vi "Prepare Log.vi"(8 "error in (no error)":errorcluster, 10 "Log":string, 11 "Log Manager Module in":refnum<class "Log Manager Module.lvclass">) -> (0 "error out":errorcluster, 3 "Log Manager Module out":refnum<class "Log Manager Module.lvclass">)   [LabVIEW 2020, in "VolatusData.lvlib" / "Log Manager Module.lvclass"]
uses:
  Log Manager Module.lvclass
  C:/dev/lv20CE/relink/lv-volatus/Volatus/Module/Module.lvclass
  Prep State.ctl
  Log Manager Module.lvclass/Log Manager Module.ctl
  <vilib>/Utility/miscctls.llb/LVMapReplaceAction.ctl
  Prep Info.ctl
  Log Preparer Module/Log Preparer Module.lvclass
  VolatusData.lvlib
  C:/dev/lv20CE/relink/lv-volatus/VolatusData/Log Manager Module/Log Manager Module.lvclass
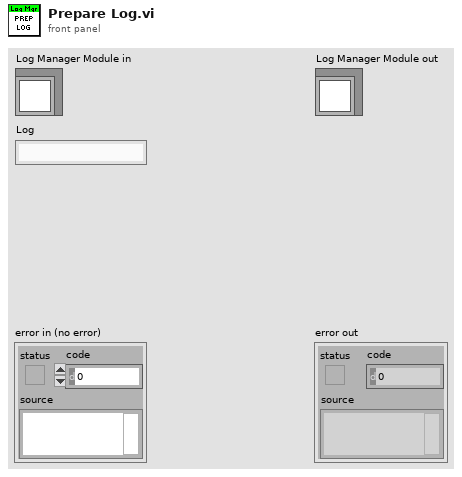
[diagram p1: front panel]
types:
  T1 = typedef "VolatusData.lvlib/Prep State.ctl" = enum16{"Unknown", "In Progress", "Success", "Failed"}
  T2 = typedef "VolatusData.lvlib/Log Manager Module.lvclass/Prep Info.ctl" = cluster{"State":T1, "Error":errorcluster}
  T3 = typedef "LVMapReplaceAction.ctl" = enum32{"Modify Entry only if found", "Add or Modify Entry", "Delete Entry"}
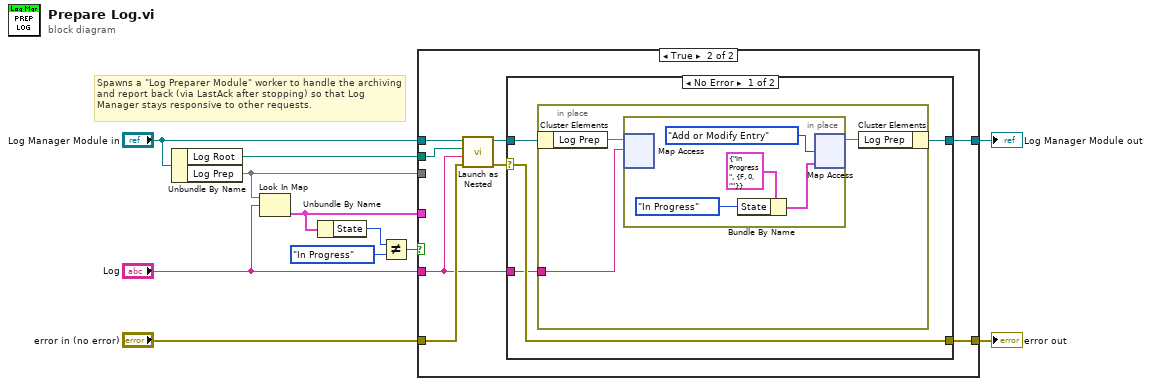
[diagram p0: block diagram]
diagram:
  # "Spawns a \"Log Preparer Module\" worker to handle the archiving and report back (via LastAck after stopping) so that Log Manager stays responsive to other requests."
  n1 = Unbundle By Name("Log Manager Module in") -> ("Log Root"=w11:path, "Log Prep"=w1:map{string, T2})
  n2 = Look In Map(map=w1, key="Log") -> (value=w2:T2)  [unwired: 1 in, 1 out]
  n3 = Unbundle By Name(w2) -> ("State"=w5:T1)
  n4 = Not Equal?(x=w5, y=Prep_State."In Progress" ("x")) -> (x != y?=w3:bool)
  n5 = case shown="True" w3 {
    tunnel: w11 -> [_ w21]
    tunnel: "Log Manager Module in" -> [w12 w20]
    tunnel: "error in (no error)" -> [w13 w19]
    tunnel: "Log" -> [_ w16]
    tunnel: [w13 w14] -> w7
    tunnel: [w12 w15] -> w6
    tunnel: w2 -> [_ _]
    tunnel: w1 -> [_ _]
    frame False {
      # "Log already being processed"
    }
    frame True {
      n6 = call "Launch as Nested.vi"("error in (no error)"=w19, "Log"=w16, "Log Root"=w21, "Parent in"=w20) -> ("error out"=w18:errorcluster, "Parent"=w17:refnum<class "Log Manager Module.lvclass">)  [unwired: 5 in, 1 out]
      n7 = case shown="No Error" w18 {
        selector: w18 -> [w25 w33]
        tunnel: w17 -> [w24 w34]
        tunnel: w16 -> [w23 _]
        tunnel: [w22 w34] -> w15
        tunnel: [w25 w33] -> w14
        frame No Error {
          n8 = in-place {
            in-place-border: w23 -> [w27]
            n9 = in-place-cluster #1(w24) -> ("Log Prep"=w28:map{string, T2})
            n10 = in-place {
              n11 = in-place-map #2(w28, w27) -> ()  [unwired: 1 in, 2 out]
              n12 = Bundle By Name(cluster=T2 {"State"=enum."In Progress", "Error"={"status"=FALSE, "code"=0, "source"=""}} ("value"), "State"=Prep_State."In Progress") -> (w29:T2)
              n13 = in-place-map #2(w29, LVMapReplaceAction."Add or Modify Entry" ("action")) -> (w26:map{string, T2})  [unwired: 2 out]
            }
            n14 = in-place-cluster #1("Log Prep"=w26) -> (w22:refnum<class "Log Manager Module.lvclass">)
          }
        }
        frame Error {
        }
      }
    }
  }
  "error out" <- w7
  "Log Manager Module out" <- w6
